vi "Create.vi"(9 "Alias":string, 10 "Actor":refnum<class "Actor.lvclass">, 11 "jettl in":refnum<class "jettl.lvclass">) -> (3 "jettl out":refnum<class "jettl.lvclass">)   [LabVIEW 2021, in "jettl.lvlib" / "jettl.lvclass"]
uses:
  jettl.lvclass
  C:/git/jettl/src/jettl/Actor/Actor.lvclass
  Actor/Actor.lvclass
  State/Msg State/Msg State.lvclass
  C:/git/jettl/src/jettl/jettl/State/State/State.lvclass
  jettl.lvclass/jettl.ctl
  Actor/Loop.vi
  jettl.lvlib
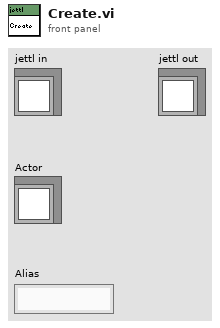
[diagram p1: front panel]
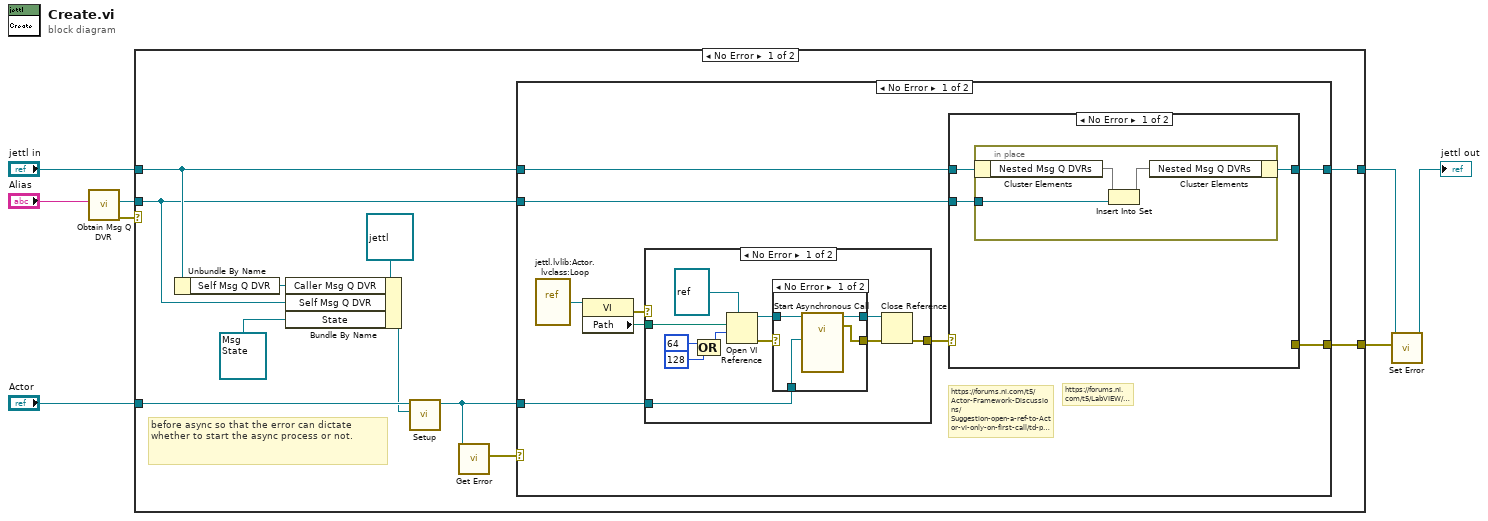
[diagram p0: block diagram]
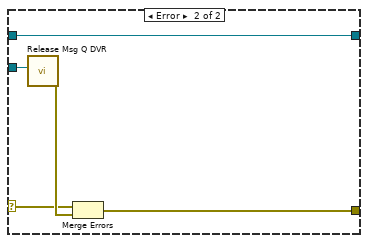
[diagram p4: hidden frame]
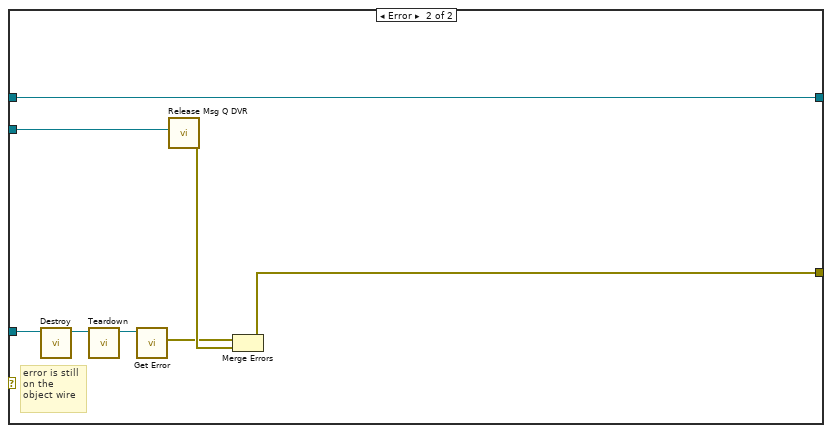
[diagram p5: hidden frame]
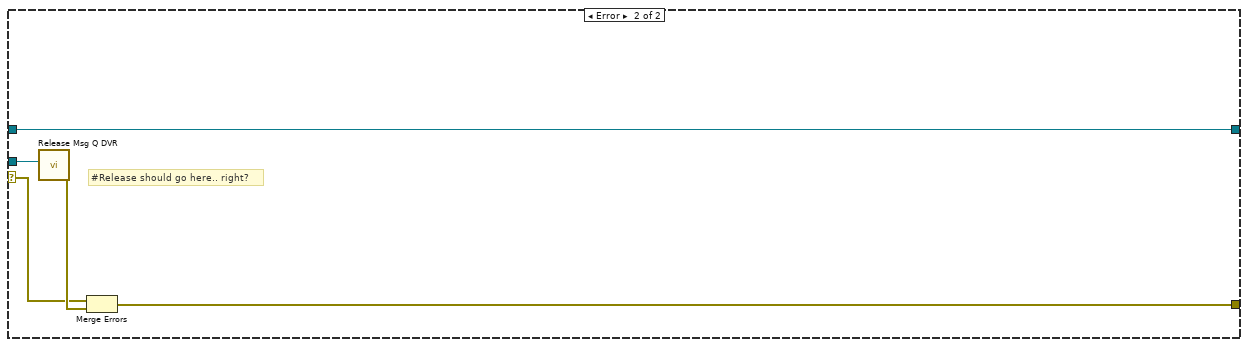
[diagram p6: hidden frame]
diagram:
  n1 = call "Obtain Msg Q DVR.vi"("Msg Q DVR Alias"="Alias") -> ("error out"=w4:errorcluster, "Msg Q DVR"=w6:refnum<data-value>)  [unwired: 9 in]
  n2 = case shown="No Error" w4 {
    selector: w4 -> [_ w66]
    tunnel: [w19 w70] -> w3
    tunnel: [w18 w68] -> w1
    tunnel: "Actor" -> [w16 _]
    tunnel: w6 -> [w13 w69]
    tunnel: "jettl in" -> [w15 w70]
    frame No Error {
      # "before async so that the error can dictate whether to start the async process or not."
      n3 = Unbundle By Name(w15) -> ("Self Msg Q DVR"=w14:refnum<data-value>)
      n4 = Bundle By Name(cluster=refnum<class "jettl.lvclass"> refnum ("Self Actor in"), "Caller Msg Q DVR"=w14, "Self Msg Q DVR"=w13, "State"=refnum<class "Msg State.lvclass"> refnum ("LVCAM.lvlib:Msging Self Actor State.lvclass")) -> (w12:refnum<class "jettl.lvclass">)
      n5 = call-dynamic "Setup.vi"("Actor"=w12, "Actor in"=w16) -> ("Actor out"=w9:refnum<class "Actor.lvclass">)  [unwired: 9 in]
      n6 = call-dynamic "Get Error.vi"("Actor in"=w9) -> ("Error"=w10:errorcluster)  [unwired: 10 in]
      n7 = case shown="No Error" w10 {
        tunnel: [w28 w64] -> w19
        tunnel: w9 -> [w27 w62]
        tunnel: [w26 w63] -> w18
        tunnel: w15 -> [w24 w64]
        tunnel: w13 -> [w23 w65]
        frame No Error {
          # "https://forums.ni.com/t5/LabVIEW/Static-VI-Reference/m-p/3334014#M978333"
          # "https://forums.ni.com/t5/Actor-Framework-Discussions/Suggestion-open-a-ref-to-Actor-vi-only-on-first-call/td-p/3451643/page/4"
          n8 = vi-ref "jettl.lvlib:Actor.lvclass:Loop.vi"() -> (w21:refnum<vi>)
          n9 = property class="VI"(reference=w21) -> (error out=w22:errorcluster, "Path"=w20:path)  [unwired: 1 in, 1 out]
          n10 = case shown="No Error" w22 {
            selector: w22 -> [_ w46]
            tunnel: [w37 w46] -> w25
            tunnel: w20 -> [w33 _]
            tunnel: w27 -> [w29 _]
            frame No Error {
              n11 = Compound Arithmetic op=OR(64 ("options: Multiple Clones,\n  Fire & Forget"), 128 ("options: Multiple Clones,\n  Fire & Forget")) -> (w35:i32)
              n12 = Open VI Reference(type specifier VI Refnum (for type only)=refnum<vi> refnum, vi path=w33, options=w35) -> (vi reference=w31:refnum<vi>, error out=w32:errorcluster)  [unwired: 3 in]
              n13 = case shown="No Error" w32 {
                selector: w32 -> [_ w45]
                tunnel: [w43 w44] -> w39
                tunnel: [w42 w45] -> w38
                tunnel: w31 -> [w41 w44]
                tunnel: w29 -> [w40 _]
                frame No Error {
                  n14 = call-by-ref "Start Asynchronous Call"(reference=w41, "Actor in"=w40) -> (reference out=w43:refnum<vi>, error out=w42:errorcluster)  [unwired: 12 in]
                }
                frame Error {
                }
              }
              n15 = Close Reference(reference=w39, error in (no error)=w38) -> (error out=w37:errorcluster)
            }
            frame Error {
            }
          }
          n16 = case shown="No Error" w25 {
            selector: w25 -> [_ w53]
            tunnel: w24 -> [w49 w57]
            tunnel: [w48 w57] -> w28
            tunnel: w23 -> [w47 w56]
            tunnel: [_ w55] -> w26
            frame No Error {
              n17 = in-place {
                in-place-border: w47 -> [w50]
                n18 = in-place-cluster #1(w49) -> ("Nested Msg Q DVRs"=w52:set{refnum<data-value>})
                n19 = Insert Into Set(10:w50, 11:w52) -> (3:w51:set{refnum<data-value>})  [unwired: 1 out]
                n20 = in-place-cluster #1("Nested Msg Q DVRs"=w51) -> (w48:refnum<class "jettl.lvclass">)
              }
            }
            frame Error {
              n21 = call "Release Msg Q DVR.vi"("Msg Q DVR"=w56) -> ("error out"=w54:errorcluster)  [unwired: 10 in]
              n22 = Merge Errors(w53, w54) -> (w55:errorcluster)
            }
          }
        }
        frame Error {
          # "error is still on the object wire"
          n23 = call-dynamic "Destroy.vi"("Destroy in"=w62) -> ("Destroy out"=w61:refnum<class "Actor.lvclass">)  [unwired: 10 in]
          n24 = call-dynamic "Teardown.vi"("Actor in"=w61) -> ("Actor out"=w60:refnum<class "Actor.lvclass">)  [unwired: 9 in, 1 out]
          n25 = call-dynamic "Get Error.vi"("Actor in"=w60) -> ("Error"=w58:errorcluster)  [unwired: 10 in]
          n26 = call "Release Msg Q DVR.vi"("Msg Q DVR"=w65) -> ("error out"=w59:errorcluster)  [unwired: 10 in]
          n27 = Merge Errors(w58, w59) -> (w63:errorcluster)
        }
      }
    }
    frame Error {
      # "#Release should go here.. right?"
      n28 = call "Release Msg Q DVR.vi"("Msg Q DVR"=w69) -> ("error out"=w67:errorcluster)  [unwired: 10 in]
      n29 = Merge Errors(w66, w67) -> (w68:errorcluster)
    }
  }
  n30 = call-dynamic "Set Error.vi"("Error"=w1, "jettl in"=w3) -> ("jettl out"=→"jettl out":refnum<class "jettl.lvclass">)  [unwired: 9 in]
